vi "NFC_TCPIP.vi"(9 "port":u16=33000, 10 "IP":string="192.168.0.79") -> (1 "Read Data":string, 2 "UID":string)   [LabVIEW 2017]
panel:
  in  "Read":string="RD_01_00000_0015"
  out "Response":string
  out "Init 2":string
  out "Init":string
  in  "Init":string="CU_00_00_00_00_00_AS"
  in  "configure channel":string="CI_01_11_0000_004_064_01_01_00"
  out "无错误":errorcluster
  in  "错误输入（无错误）":errorcluster
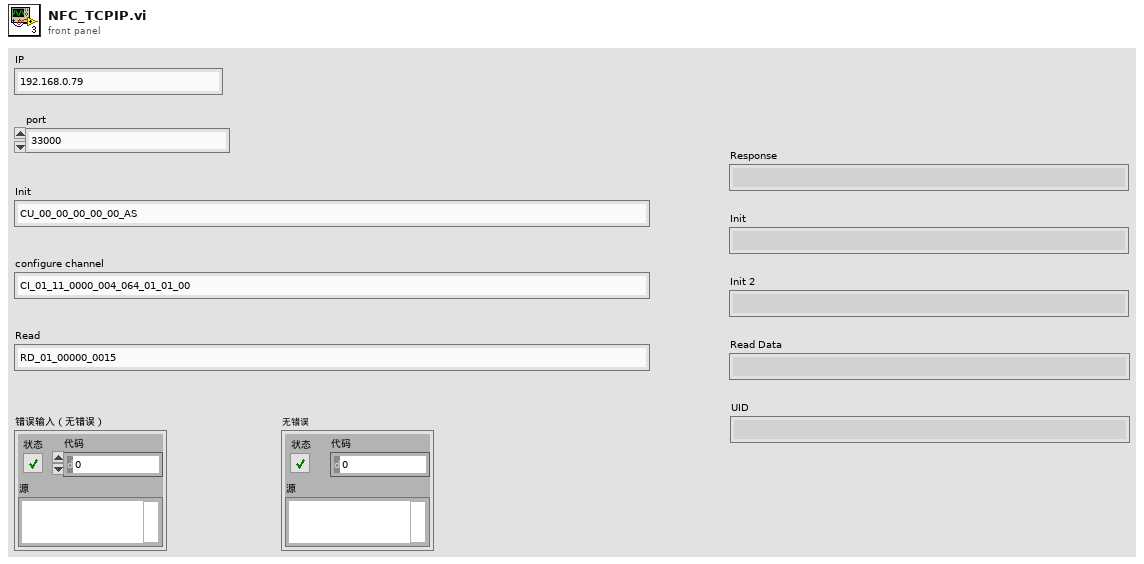
[diagram p1: front panel]
types:
  T1 = cluster{"Check UID":string, "NFC tag memory blocks 00 – 31":string, "NFC tag memory blocks 32 – 63":string, "Read Fixture ID":string, "Read UID":string, "Read Memory block":string, "Read Block size":string, "Read user data and verify bocks 00 - 31":string, "Read user data and verify bocks 32 - 63":string, "Memory secured by disabling the write access":string, "Verify the memory is secured":string, "Read user data and verify the memory (256 bytes) ":string}
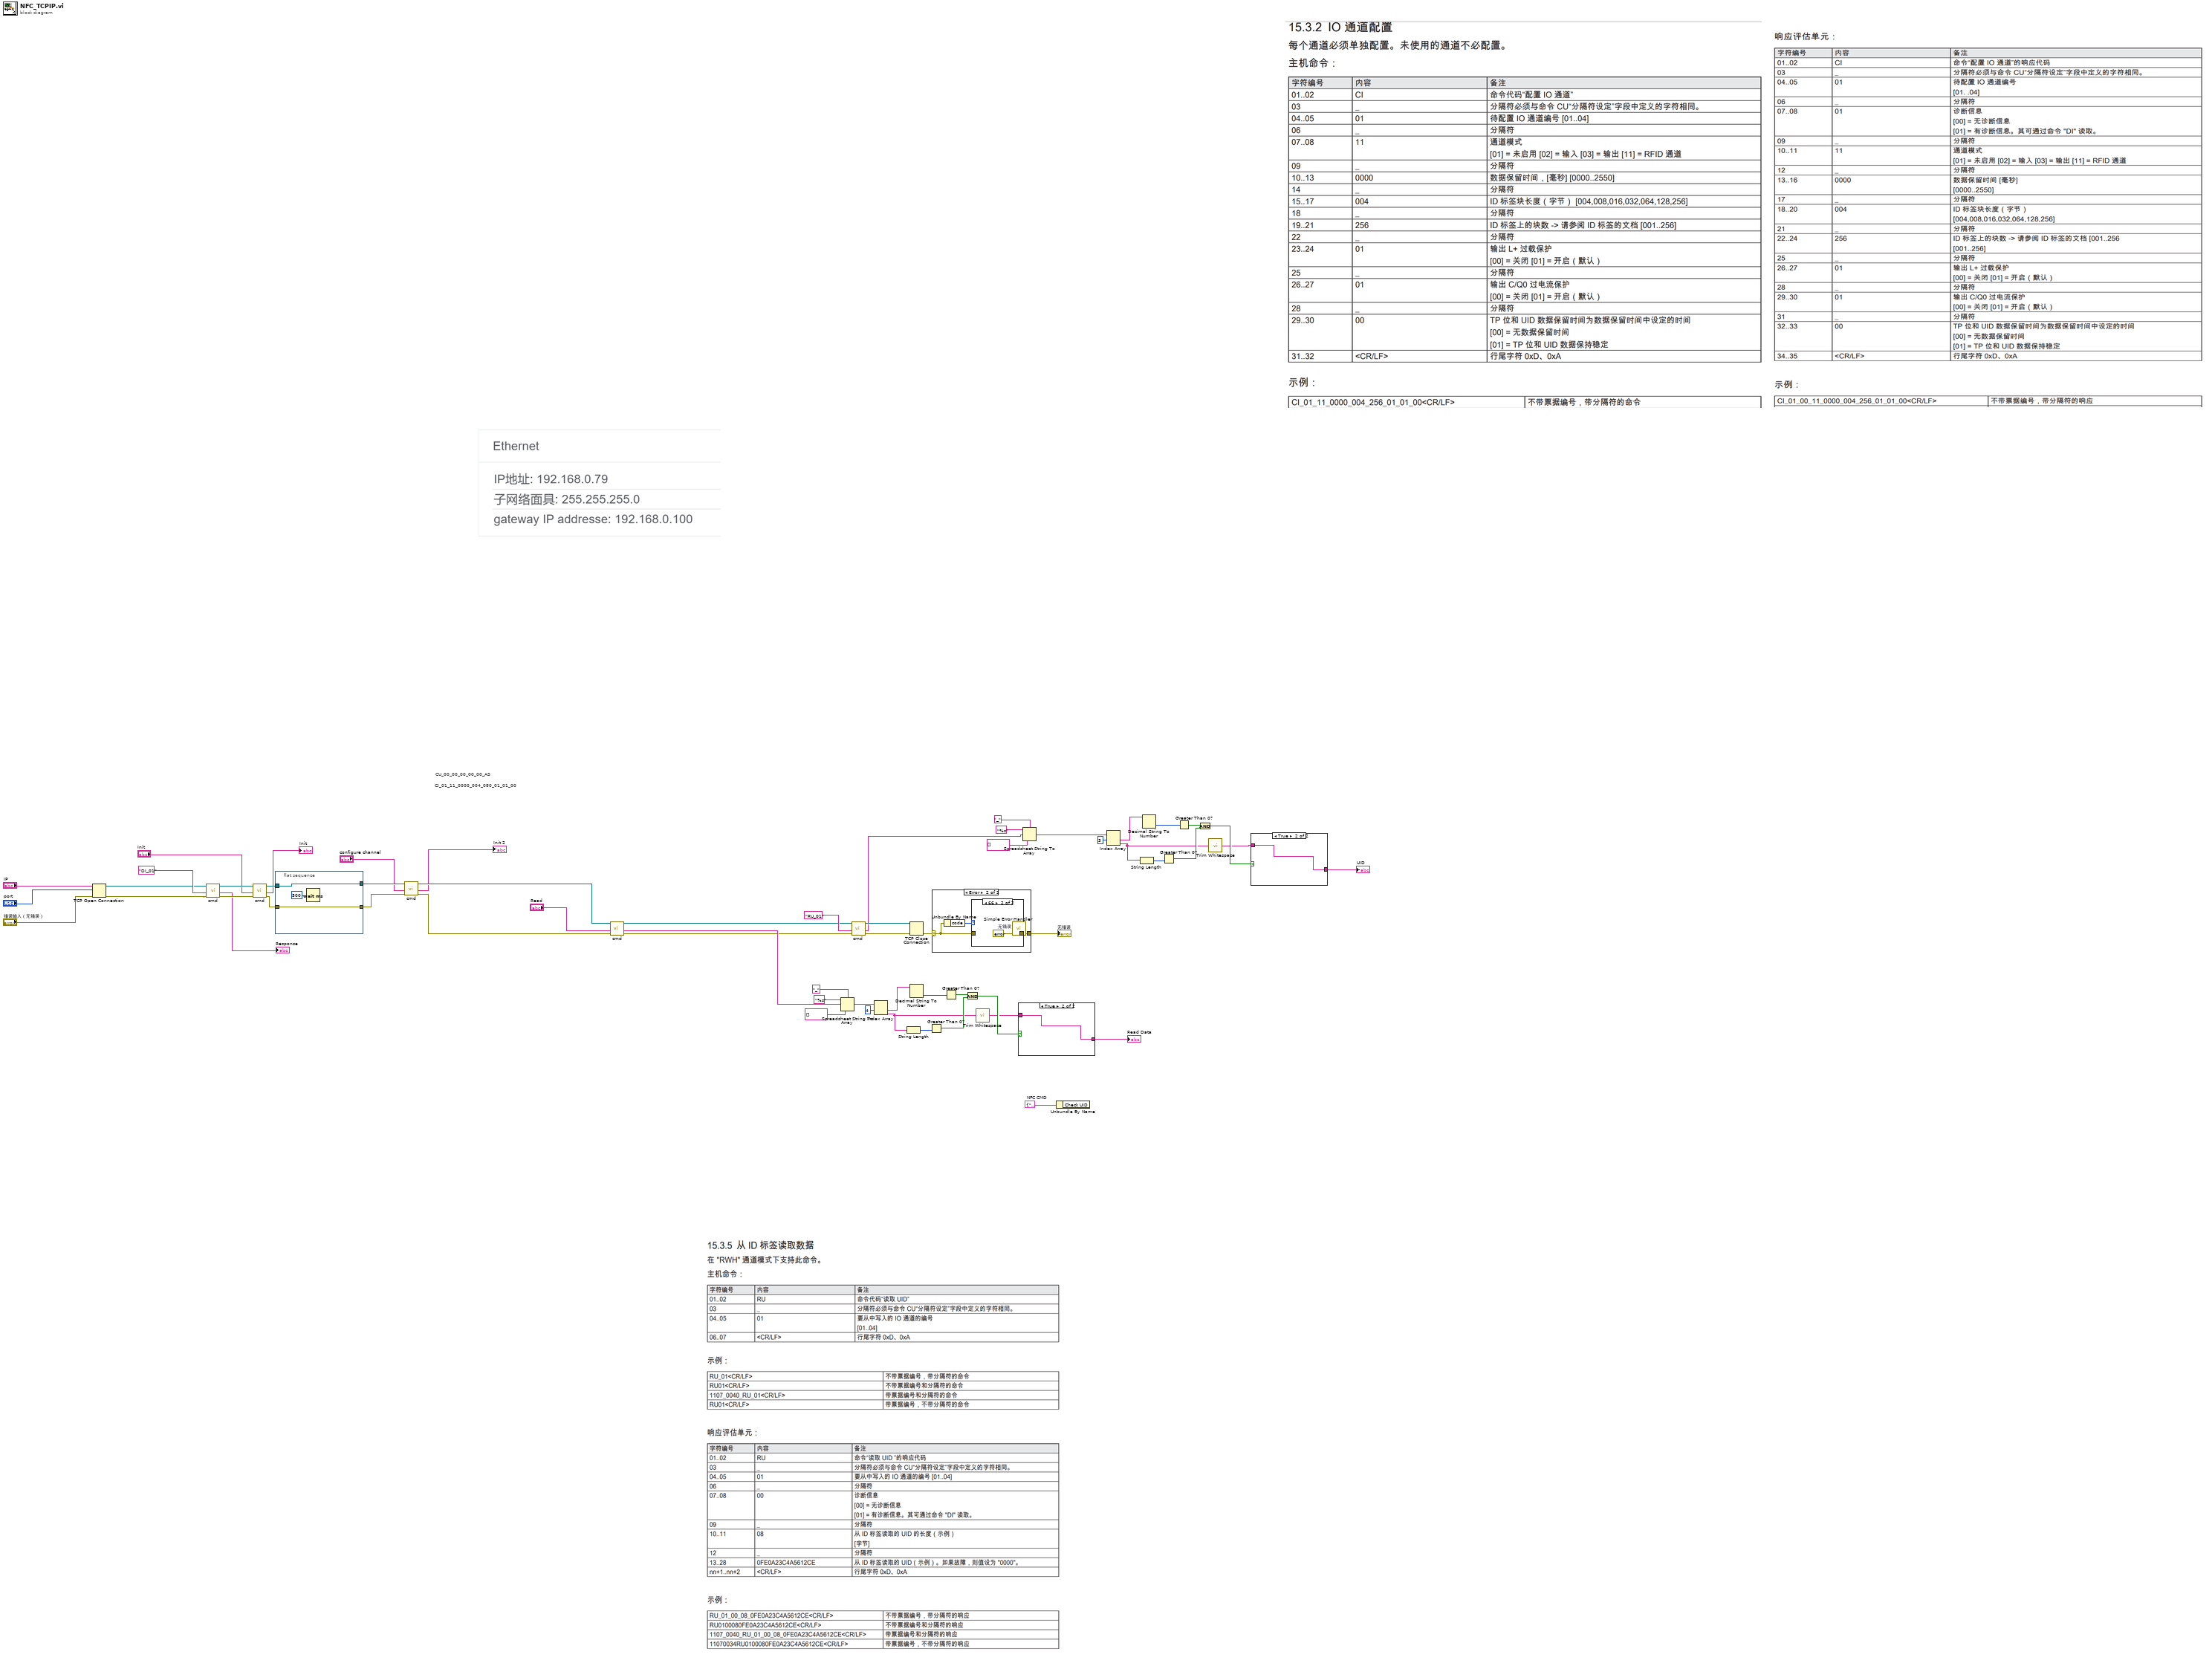
[diagram p0: block diagram]
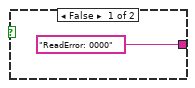
[diagram p2: hidden frame]
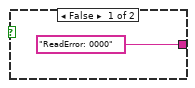
[diagram p3: hidden frame]
diagram:
  w47 = T1 {"Check UID"="ACCESSORY_TAG_READ_DATA_REQ", "NFC tag memory blocks 00 – 31"="ACCESSORY_PROGRAM_CMD", "NFC tag memory blocks 32 – 63"="TBA", "Read Fixture ID"="TBA", "Read UID"="TBA", "Read Memory block"="TBA", "Read Block size"="TBA", "Read user data and verify bocks 00 - 31"="ACCESSORY_TAG_READ_DATA_REQ", "Read user data and verify bocks 32 - 63"="TBA", "Memory secured by disabling the write access"="TBA", "Verify the memory is secured"="TBA", "Read user data and verify the memory (256 bytes) "="ACCESSORY_TAG_READ_DATA_REQ"}  # NFC CMD
  # "CI_01_11_0000_004_080_01_01_00"
  # "CU_00_00_00_00_00_AS"
  n1 = TCP Open Connection(address="IP", remote port or service name="port", error in (no error)="错误输入（无错误）") -> (connection ID=w18:refnum<k5>, error out=w17:errorcluster)  [unwired: 2 in]
  n2 = call "cmd.vi"("错误输入"=w17, "Cmd"="DI_01", "连接ID"=w18) -> ("错误输出"=w37:errorcluster, "Response"=→"Response":string, "连接ID输出"=w38:refnum<k5>)  [unwired: 6 in]
  n3 = call "cmd.vi"("错误输入"=w37, "Cmd"="Init", "连接ID"=w38) -> ("错误输出"=w45:errorcluster, "Response"=→"Init":string, "连接ID输出"=w46:refnum<k5>)  [unwired: 6 in]
  n4 = flat-sequence {
    tunnel: w45 -> [w60]
    tunnel: [w60] -> w43
    tunnel: w46 -> [w59]
    tunnel: [w59] -> w44
    frame #0 {
      n5 = Wait (ms)(milliseconds to wait=u32 500 ("等待时间（毫秒）")) -> ()  [unwired: 1 out]
    }
  }
  n6 = call "cmd.vi"("错误输入"=w43, "Cmd"="configure channel", "连接ID"=w44) -> ("错误输出"=w26:errorcluster, "Response"=→"Init 2":string, "连接ID输出"=w42:refnum<k5>)  [unwired: 6 in]
  n7 = call "cmd.vi"("错误输入"=w26, "Cmd"="Read", "连接ID"=w42) -> ("错误输出"=w21:errorcluster, "Response"=w41:string, "连接ID输出"=w22:refnum<k5>)  [unwired: 6 in]
  n8 = Spreadsheet String To Array(delimiter (Tab)="_" ("分隔符(Tab)"), format string="%s" ("格式字符串"), spreadsheet string=w41, array type (2D Dbl)=string[] []) -> (array=w50:string[])
  n9 = call "cmd.vi"("错误输入"=w21, "Cmd"="RU_01", "连接ID"=w22) -> ("错误输出"=w19:errorcluster, "Response"=w13:string, "连接ID输出"=w20:refnum<k5>)  [unwired: 6 in]
  n10 = Index Array(array=w50, index #1=4 ("索引")) -> (element #1=w33:string, element #2=w25:string)  [unwired: 1 in]
  n11 = String Length(string=w25) -> (length=w28:i32)
  n12 = Decimal String To Number(string=w33) -> (number=w32:i32)  [unwired: 2 in, 1 out]
  n13 = TCP Close Connection(connection ID=w20, error in (no error)=w19) -> (error out=w57:errorcluster)  [unwired: 1 in, 1 out]
  n14 = Greater Than 0?(x=w28) -> (x > 0?=w30:bool)
  n15 = case shown="Error" w57 {
    selector: w57 -> [w62 w64]
    tunnel: [w62 w63] -> w56
    frame No Error {
    }
    frame Error {
      n16 = Unbundle By Name(w64) -> ("code"=w65:i32)
      n17 = case shown="66" w65 {
        tunnel: w64 -> [w66 _]
        tunnel: [w66 w67] -> w63
        frame Default {
        }
        frame 66 {
          w67 = errorcluster {"status"=FALSE, "code"=0, "source"=""}  # 无错误
        }
      }
    }
  }
  "无错误" <- w56
  n18 = Greater Than 0?(x=w32) -> (x > 0?=w31:bool)
  n19 = And(x=w31, y=w30) -> (x .and. y?=w29:bool)
  n20 = call <vilib>:"Trim Whitespace.vi"("string"=w25) -> ("trimmed string"=w24:string)  [unwired: 1 in]
  n21 = call <vilib>:"Simple Error Handler.vi"("error in (no error)"=w56) -> ()  [unwired: 4 in, 5 out]
  n22 = case shown="True" w29 {
    tunnel: ["ReadError: 0000" ("y") w69] -> w48
    tunnel: w24 -> [_ w69]
    frame False {
    }
    frame True {
    }
  }
  "Read Data" <- w48
  n23 = Spreadsheet String To Array(delimiter (Tab)="_" ("分隔符(Tab)"), format string="%s" ("格式字符串"), spreadsheet string=w13, array type (2D Dbl)=string[] []) -> (array=w2:string[])
  n24 = Unbundle By Name(w47) -> ()  [unwired: 1 out]
  n25 = Index Array(array=w2, index #1=3 ("索引")) -> (element #1=w11:string, element #2=w5:string)  [unwired: 1 in]
  n26 = String Length(string=w5) -> (length=w6:i32)
  n27 = Decimal String To Number(string=w11) -> (number=w10:i32)  [unwired: 2 in, 1 out]
  n28 = Greater Than 0?(x=w6) -> (x > 0?=w8:bool)
  n29 = Greater Than 0?(x=w10) -> (x > 0?=w9:bool)
  n30 = And(x=w9, y=w8) -> (x .and. y?=w7:bool)
  n31 = call <vilib>:"Trim Whitespace.vi"("string"=w5) -> ("trimmed string"=w4:string)  [unwired: 1 in]
  n32 = case shown="True" w7 {
    tunnel: ["ReadError: 0000" ("y") w71] -> w1
    tunnel: w4 -> [_ w71]
    frame False {
    }
    frame True {
    }
  }
  "UID" <- w1
